vi "HW Config_Check if HW Parameters are OK.vi"(11 "HW Configuration (each Station)":T1={"Results FilePath"=path "", "Analysis Parameters"={"Area"={"Lower Value"=10.0, "Upper Value"=500.0}, "Circle Filter Radius"={"Lower Value"=10.0, "Upper Value"=500.0}, "Edge Detection Threshold"=50}, "ROI Parameters"={"ROI size (in Radius)"={"Width"=1.0, "Height"=0.5}}}) -> (2 "Info OK?":bool, 3 "HW Configuration (each Station)":T1={"Results FilePath"=path "", "Analysis Parameters"={"Area"={"Lower Value"=10.0, "Upper Value"=500.0}, "Circle Filter Radius"={"Lower Value"=10.0, "Upper Value"=500.0}, "Edge Detection Threshold"=50}, "ROI Parameters"={"ROI size (in Radius)"={"Width"=1.0, "Height"=0.5}}})   [LabVIEW 2014]
uses:
  Custom Controls/TypeDef - System Configuration.ctl
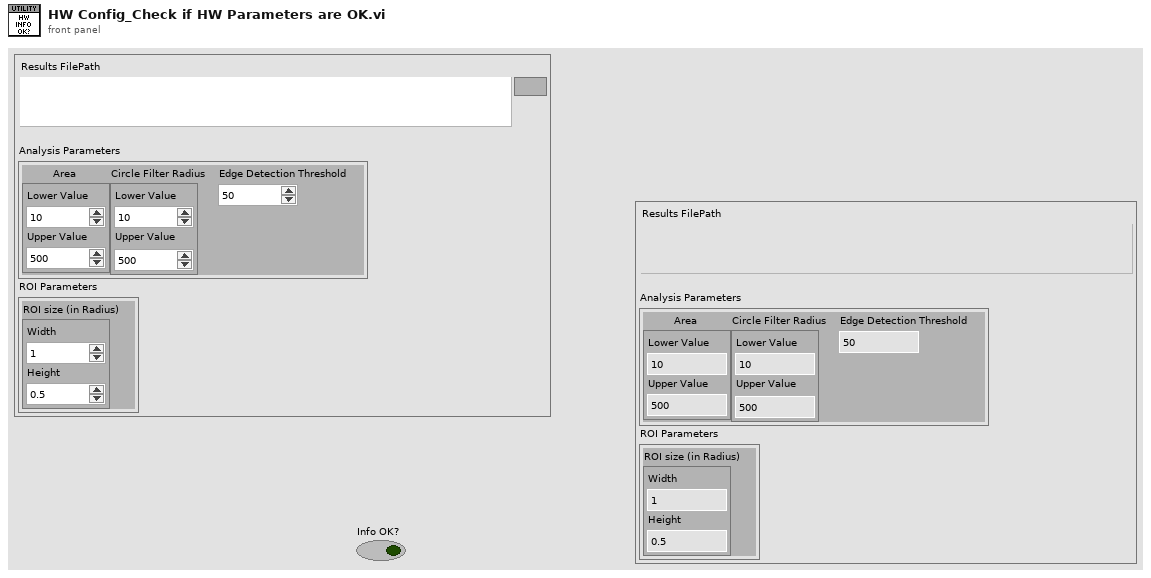
[diagram p1: front panel]
types:
  T1 = typedef "TypeDef - System Configuration.ctl" = cluster{"Results FilePath":path, "Analysis Parameters":cluster{"Area":cluster{"Lower Value":dbl, "Upper Value":dbl}, "Circle Filter Radius":cluster{"Lower Value":sgl, "Upper Value":sgl}, "Edge Detection Threshold":u16}, "ROI Parameters":cluster{"ROI size (in Radius)":cluster{"Width":dbl, "Height":dbl}}}
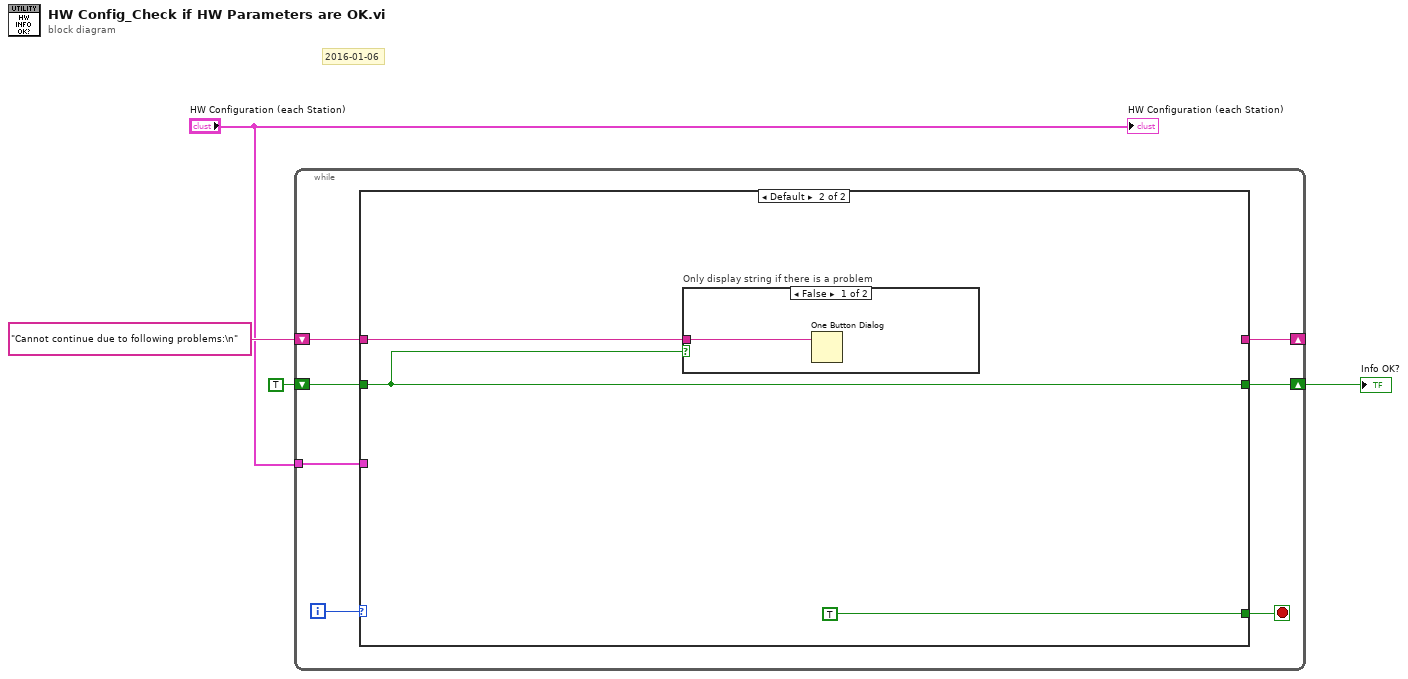
[diagram p0: block diagram]
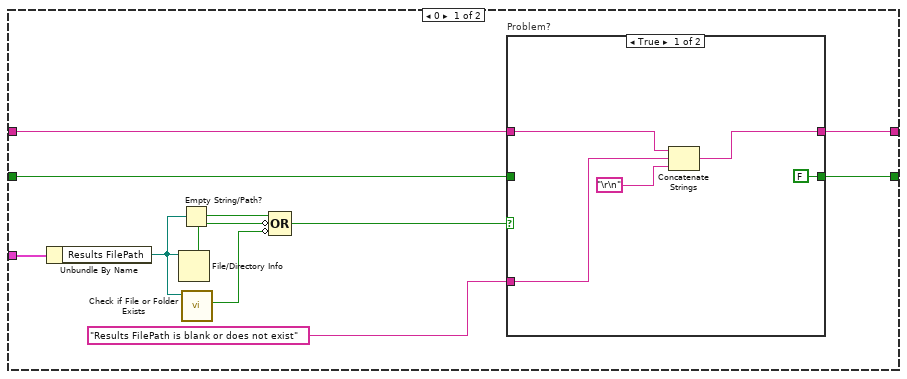
[diagram p2: hidden frame]
diagram:
  # "2016-01-06"
  n1 = while {
    shift-right: [w8] -> w4
    shift-left: TRUE -> [w9]
    shift-right: [w5] -> _
    shift-left: "Cannot continue due to following problems:\n" -> [w7]
    tunnel: "HW Configuration (each Station)" -> [w6]
    i -> [w11]
    stop <- w10 stop-if-true
    n2 = case shown="Default" w11 {
      tunnel: [_ TRUE] -> w10
      tunnel: w9 -> [w19 w31]
      tunnel: [w20 w31] -> w8
      tunnel: w7 -> [w21 w30]
      tunnel: w6 -> [w17 _]
      tunnel: [w22 _] -> w5
      frame 0 {
        n3 = Unbundle By Name(w17) -> ("Results FilePath"=w13:path)
        n4 = File/Directory Info(path=w13) -> (directory=w14:bool)  [unwired: 1 in, 6 out]
        n5 = Empty String/Path?(string/path=w13) -> (empty?=w16:bool)
        n6 = call <vilib>:"Check if File or Folder Exists.vi"("path"=w13) -> ("file or folder exists?"=w12:bool)  [unwired: 8 in, 2 out]
        n7 = Compound Arithmetic op=OR(w16, invert w14, invert w12) -> (w15:bool)
        n8 = case "Problem?" shown="True" w15 {
          tunnel: [w25 w29] -> w22
          tunnel: w21 -> [w26 w29]
          tunnel: [FALSE w28] -> w20
          tunnel: w19 -> [_ w28]
          tunnel: "Results FilePath is blank or does not exist" -> [w24 _]
          frame True {
            n9 = Concatenate Strings(w26, w24, "\r\n") -> (w25:string)
          }
          frame False {
          }
        }
      }
      frame Default {
        n10 = case "Only display string if there is a problem" shown="False" w31 {
          tunnel: w30 -> [w33 _]
          frame False {
            n11 = One Button Dialog(message=w33) -> ()  [unwired: 1 in, 1 out]
          }
          frame True {
          }
        }
      }
    }
  }
  "Info OK?" <- w4
  "HW Configuration (each Station)" <- "HW Configuration (each Station)"
